vi "Replicate Hierarchy.vi"(0 "Root Path":path, 5 "Destination Path":path, 11 "error in (no error)":errorcluster) -> (4 "Replicated Hierarchy":path[](array[path]), 15 "error out":errorcluster)   [LabVIEW 2011]
doc: "Replicates a folder of files to a new location and maintains hierarchy. This VI was provided by the Systems Engineering group at NI.\n\nAAL 9/09"
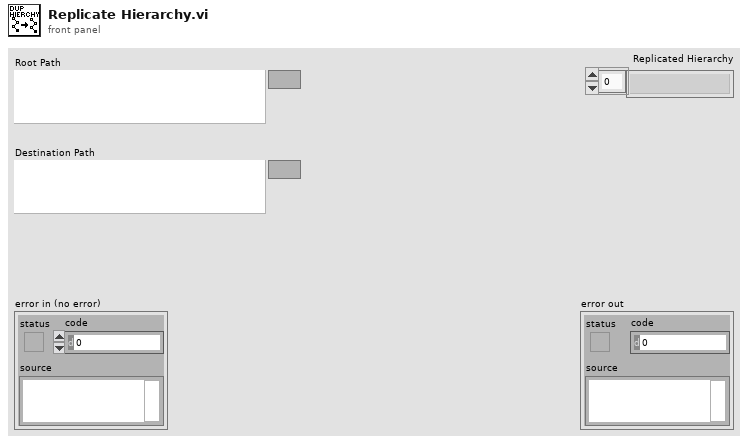
[diagram p1: front panel]
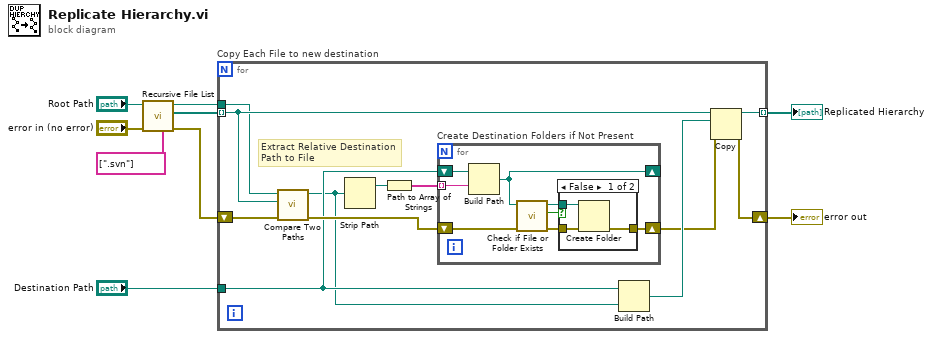
[diagram p0: block diagram]
diagram:
  n1 = call <vilib>:"Recursive File List.vi"("Folders to Exclude"=string[] [".svn"], "error in (no error)"="error in (no error)", "Folder Path"="Root Path") -> ("error out"=w7:errorcluster, "All Files in Dir"=w2:path[], "dup Folder Path"=w9:path)  [unwired: 1 in, 5 out]
  n2 = for "Copy Each File to new destination" {
    tunnel: w2 -> [w19] mode=indexing
    tunnel: "Destination Path" -> [w15]
    tunnel: [w20] -> w4 mode=indexing
    shift-right: [w11] -> w8
    shift-left: w7 -> [w13]
    tunnel: w9 -> [w10]
    # "Extract Relative Destination Path to File"
    n3 = call <vilib>:"Compare Two Paths.vi"("error in (no error)"=w13, "Path 2"=w19, "Path 1"=w10) -> ("error out"=w21:errorcluster, "Relative Path from 1 to 2"=w14:path)  [unwired: 7 out]
    n4 = Strip Path(path=w14) -> (stripped path=w17:path)  [unwired: 1 out]
    n5 = Path to Array of Strings(0:w17) -> (2:w16:string[])  [unwired: 1 out]
    n6 = for "Create Destination Folders if Not Present" {
      tunnel: w16 -> [w29] mode=indexing
      shift-right: [w27] -> _
      shift-left: w15 -> [w28]
      shift-right: [w22] -> w12
      shift-left: w21 -> [w24]
      n7 = Build Path(base path=w28, name or relative path=w29) -> (appended path=w27:path)
      n8 = call <vilib>:"Check if File or Folder Exists.vi"("error in (no error)"=w24, "path"=w27) -> ("error out"=w23:errorcluster, "file or folder exists?"=w26:bool, "dup path"=w25:path)  [unwired: 7 out]
      n9 = case shown="False" w26 {
        tunnel: w25 -> [w32 _]
        tunnel: w23 -> [w31 w33]
        tunnel: [w30 w33] -> w22
        frame False {
          n10 = Create Folder(path (use dialog)=w32, error in=w31) -> (error out=w30:errorcluster)  [unwired: 3 out]
        }
        frame True {
        }
      }
    }
    n11 = Build Path(base path=w15, name or relative path=w14) -> (appended path=w18:path)
    n12 = Copy(8:w12, 10:w18, 11:w19) -> (0:w11:errorcluster, 3:w20:path)  [unwired: 3 out]
  }
  "error out" <- w8
  "Replicated Hierarchy" <- w4
